vi "Receptor SERIALvi.vi"() -> ()   [LabVIEW 2020]
uses:
  <vilib>/Instr/_visa.llb/VISA Configure Serial Port (Instr).vi
panel:
  out "DATA RX":string
  in  "DATA TX":string
  in  "ConfigSerial":T1={"baud rate (9600)"=9600, "data bits (8)"=8, "parity (0:none)"=enum."None", "stop bits (10: 1 bit)"=10, "flow control (0:none)"=0, "VISA resource name"="", "error in (no error) 2"={"status"=FALSE, "code"=0, "source"=""}} {"flow control (0:none)" items=["None", "XON/XOFF", "RTS/CTS", "XON/XOFF & RTS/CTS", "DTR/DSR", "XON/XOFF & DTR/DSR"]; "stop bits (10: 1 bit)" items=["1.0"=10, "1.5"=15, "2.0"=20]; "data bits (8)" min=5 max=8 step=1}
  in  "Stop":bool
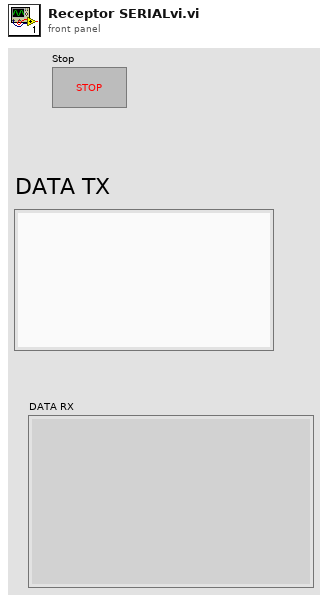
[diagram p1: front panel]
types:
  T1 = cluster{"baud rate (9600)":u32, "data bits (8)":u16, "parity (0:none)":enum16{"None", "Odd", "Even", "Mark", "Space"}, "stop bits (10: 1 bit)":u16, "flow control (0:none)":u16, "VISA resource name":refnum<visa-resource-name>, "error in (no error) 2":errorcluster}
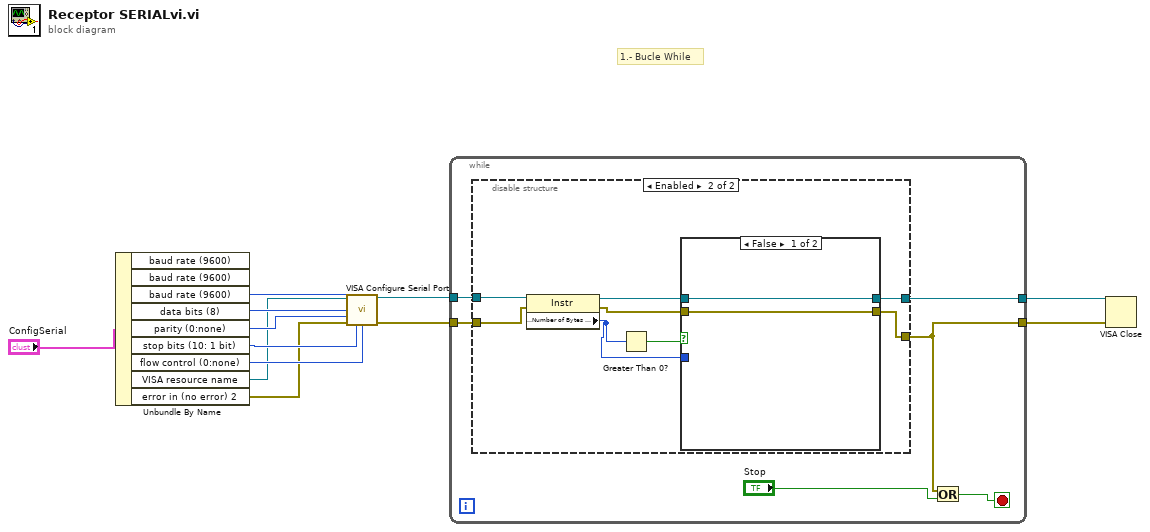
[diagram p0: block diagram]
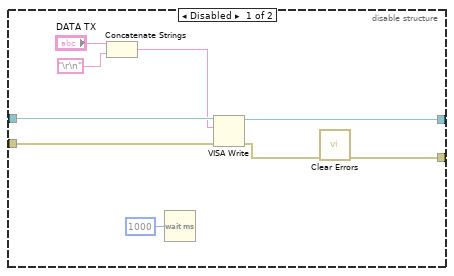
[diagram p2: hidden frame]
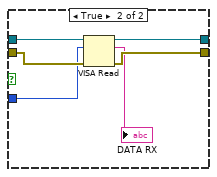
[diagram p3: hidden frame]
diagram:
  # "1.- Bucle While"
  n1 = Unbundle By Name("ConfigSerial") -> ("baud rate (9600)"=w11:u32, "data bits (8)"=w10:u16, "parity (0:none)"=w9:enum16{"None", "Odd", "Even", "Mark", "Space"}, "stop bits (10: 1 bit)"=w8:u16, "flow control (0:none)"=w7:u16, "VISA resource name"=w6:refnum<visa-resource-name>, "error in (no error) 2"=w3:errorcluster)  [unwired: 2 out]
  n2 = call-poly "VISA Configure Serial Port"("VISA resource name"=w6, "baud rate (9600)"=w11, "data bits (8)"=w10, "parity (0:none)"=w9, "error in (no error)"=w3, "stop bits (10: 1 bit)"=w8, "flow control (0:none)"=w7) -> ("VISA resource name out"=w5:refnum<visa-resource-name>, "error out"=w4:errorcluster)  [unwired: 7 in]
  n3 = while {
    tunnel: w5 -> [w18]
    tunnel: w4 -> [w17]
    tunnel: [w14] -> w2
    tunnel: [w13] -> w1
    stop <- w16 stop-if-true
    n4 = disable-structure shown="Enabled" {
      disable-tunnel: w18 -> [w27 w35]
      disable-tunnel: w17 -> [w26 w34]
      disable-tunnel: [w25 w32] -> w14
      disable-tunnel: [w22 w30] -> w13
      frame Disabled {
        n5 = Concatenate Strings("DATA TX", "\r\n") -> (w19:string)
        n6 = Wait (ms)(milliseconds to wait=u32 1000) -> ()  [unwired: 1 out]
        n7 = VISA Write(VISA resource name=w27, write buffer=w19, error in (no error)=w26) -> (VISA resource name out=w25:refnum<visa-resource-name>, error out=w23:errorcluster)  [unwired: 1 out]
        n8 = call <vilib>:"Clear Errors.vi"("error in (no error)"=w23) -> ("error out"=w22:errorcluster)  [unwired: 5 in, 1 out]
      }
      frame Enabled {
        n9 = property class="Instr"(reference=w35, error in=w34) -> (reference out=w31:refnum<visa-resource-name>, error out=w29:errorcluster, "Serial Settings:Number of Bytes at Serial Port"=w28:u32)
        n10 = Greater Than 0?(x=w28) -> (x > 0?=w33:bool)
        n11 = case shown="False" w33 {
          tunnel: [w37 w42] -> w32
          tunnel: w31 -> [w37 w43]
          tunnel: [w36 w41] -> w30
          tunnel: w29 -> [w36 w40]
          tunnel: w28 -> [_ w39]
          frame False {
          }
          frame True {
            n12 = VISA Read(VISA resource name=w43, byte count=w39, error in (no error)=w40) -> (VISA resource name out=w42:refnum<visa-resource-name>, read buffer=→"DATA RX":string, error out=w41:errorcluster)  [unwired: 1 out]
          }
        }
      }
    }
    n13 = Or(x=w13, y="Stop") -> (x .or. y?=w16:bool)
  }
  n14 = VISA Close(VISA resource name=w2, error in (no error)=w1) -> ()  [unwired: 1 out]
